vi "Mechanical Action.vi"() -> ()   [LabVIEW 2013]
doc: "该VI演示了布尔控件的机械操作。按钮值为TRUE时，指示灯点亮并且计数器值增加。按钮值为FALSE时，指示灯熄灭并且计数器值减少。所有按钮的默认状态为FALSE。\n\n共有两种布尔机械动作：转换和触发。处于转换模式时，在用户动作下，按钮将切换至默认状态。处于触发模式时，在用户动作或者按钮值被程序框图接线端读取的情况下，开关将切换至默认状态。"
panel:
  in  "机械动作":T1(radio)
  out "选项卡控件":T2(tab)
  in  "单击时转换按钮":bool
  out "单击时转换的状态":bool
  out "单击时转换的计数器":i32
  in  "释放时转换按钮":bool
  out "释放时转换的状态":bool
  out "释放时转换的计数器":i32
  in  "保持转换直到释放按钮":bool
  out "保持转换直到释放的状态":bool
  out "保持转换直到释放的计数器":i32
  in  "单击时触发按钮":bool
  out "单击时触发的状态":bool
  out "单击时触发的计数器":i32
  in  "释放时触发按钮":bool
  out "释放时触发的状态":bool
  out "释放时触发的计数器":i32
  in  "保持触发直到释放按钮":bool
  out "保持触发直到释放的计数器":i32
  out "保持触发直到释放的状态":bool
  in  "计数器清零":bool
  in  "停止":bool
  # "概述：演示布尔控件的各种机械动作。\n操作步骤：\n1. 运行VI。\n2. 选择一个机械动作对应的图片。\n3. 单击并按下按钮，查看某个机械动作的特征。\n4. 重复步骤2、3，查看其他机械动作。\n5. 单击停止停止VI。"
  # "这些选项对应于布尔控件右键菜单中的机械选项。"
  # "布尔控件有六种机械动作设置。当按钮的值为TRUE时，状态灯点亮，计数器的值递增。所有按钮的默认状态都是FALSE。机械动作有两种，一种是转换，另一种是触发。处于转换模式时，在用户动作下，按钮将切换至默认状态。处于触发模式时，在用户动作或者按钮值被程序框图接线端读取的情况下，开关将切换至默认状态。"
  # "单击时转换－按下按钮即转换状态。保持按下的状态直到按下其他按钮。"
  # "释放时转换－释放按钮时改变状态。释放其他按钮之前保持当前状态。"
  # "保持转换直到释放－按下按钮时改变状态。释放按钮时返回原状态。"
  # "单击时触发－按钮按下时转换状态。控件值被LabVIEW读取后立即恢复状态。"
  # "释放时触发－释放按钮时改变状态。控件值被LabVIEW读取后立即恢复状态。"
  # "保持触发直到释放－按下按钮时改变状态。释放按钮且LabVIEW读取控件值后返回原状态。"
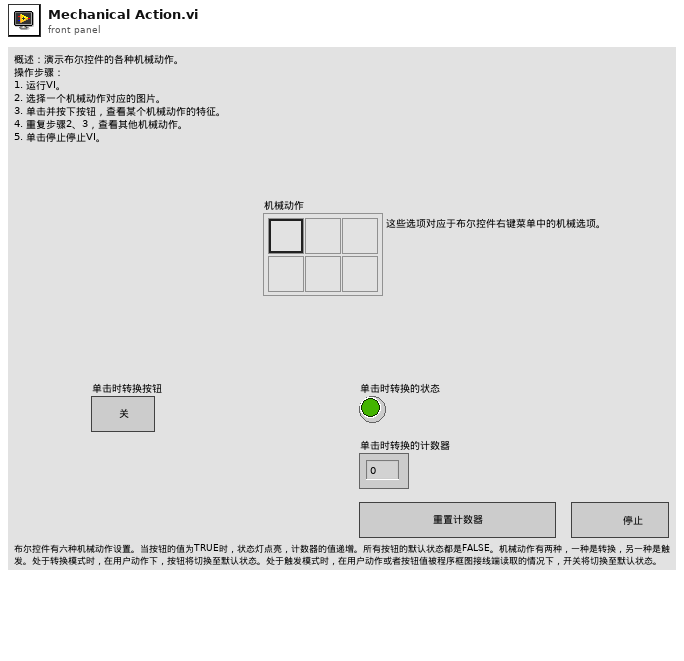
[diagram p1: front panel]
types:
  T1 = enum32{"单击时转换", "释放时转换", "保持转换直到释放", "单击时触发", "释放时触发", "保持触发直到释放"}
  T2 = enum32{"Switch When Pressed", "Switch When Released", "Switch Until Released", "Latch When Pressed", "Latch When Released", "Latch Until Released"}
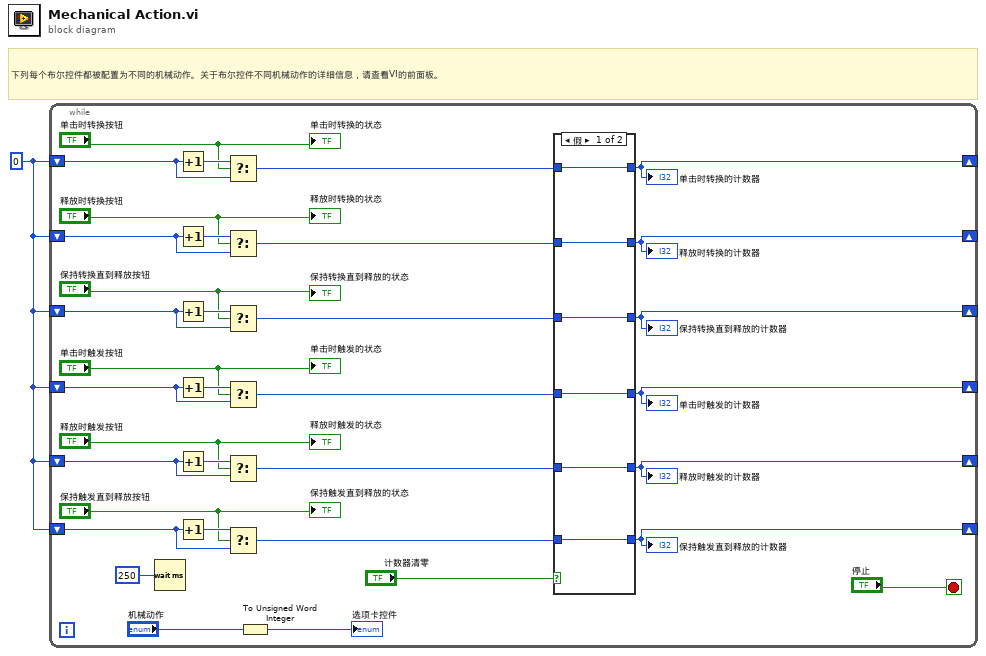
[diagram p0: block diagram]
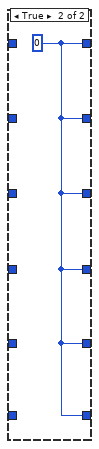
[diagram p2: hidden frame]
diagram:
  w1 = 0
  # "下列每个布尔控件都被配置为不同的机械动作。关于布尔控件不同机械动作的详细信息，请查看VI的前面板。"
  n1 = while {
    shift-left: w1 -> [w25]
    shift-right: [w12] -> _
    shift-left: w1 -> [w28]
    shift-right: [w11] -> _
    shift-left: w1 -> [w29]
    shift-right: [w10] -> _
    shift-left: w1 -> [w32]
    shift-right: [w9] -> _
    shift-left: w1 -> [w33]
    shift-right: [w8] -> _
    shift-left: w1 -> [w35]
    shift-right: [w7] -> _
    stop <- "停止" stop-if-true
    n2 = Wait (ms)(milliseconds to wait=u32 250) -> ()  [unwired: 1 out]
    n3 = Increment(x=w25) -> (x+1=w26:i32)
    n4 = Increment(x=w28) -> (x+1=w27:i32)
    n5 = Increment(x=w29) -> (x+1=w30:i32)
    n6 = Increment(x=w32) -> (x+1=w31:i32)
    n7 = Increment(x=w33) -> (x+1=w34:i32)
    n8 = Increment(x=w35) -> (x+1=w36:i32)
    n9 = Select(t=w26, s="单击时转换按钮", f=w25) -> (s? t:f=w19:i32)
    n10 = Select(t=w27, s="释放时转换按钮", f=w28) -> (s? t:f=w20:i32)
    n11 = Select(t=w30, s="保持转换直到释放按钮", f=w29) -> (s? t:f=w21:i32)
    n12 = Select(t=w31, s="单击时触发按钮", f=w32) -> (s? t:f=w22:i32)
    n13 = Select(t=w34, s="释放时触发按钮", f=w33) -> (s? t:f=w23:i32)
    n14 = Select(t=w36, s="保持触发直到释放按钮", f=w35) -> (s? t:f=w24:i32)
    n15 = To Unsigned Word Integer(number="机械动作") -> (unsigned 16bit integer=→"选项卡控件":u16)
    n16 = case shown="假" "计数器清零" {
      tunnel: [w42 w43] -> w7
      tunnel: w24 -> [w42 _]
      tunnel: [w41 w43] -> w8
      tunnel: w23 -> [w41 _]
      tunnel: [w40 w43] -> w9
      tunnel: w22 -> [w40 _]
      tunnel: [w39 w43] -> w10
      tunnel: w21 -> [w39 _]
      tunnel: [w38 w43] -> w11
      tunnel: w20 -> [w38 _]
      tunnel: [w37 w43] -> w12
      tunnel: w19 -> [w37 _]
      frame False {
      }
      frame True {
        w43 = 0
      }
    }
    "单击时转换的计数器" <- w12
    "释放时转换的计数器" <- w11
    "保持转换直到释放的计数器" <- w10
    "单击时触发的计数器" <- w9
    "释放时触发的计数器" <- w8
    "保持触发直到释放的计数器" <- w7
    "单击时转换的状态" <- "单击时转换按钮"
    "释放时转换的状态" <- "释放时转换按钮"
    "保持转换直到释放的状态" <- "保持转换直到释放按钮"
    "单击时触发的状态" <- "单击时触发按钮"
    "释放时触发的状态" <- "释放时触发按钮"
    "保持触发直到释放的状态" <- "保持触发直到释放按钮"
  }
